vi "Device Level, Display Pulses.vi"(0 "error in":errorcluster, 2 "WFGraph Refnum":refnum<vi>, 3 "waveform":waveform(dbl)={"t0"=timestamp(0 s since 1904-01-01), "dt"=nan, "Y"=[]}, 4 "Zoom (F)":bool) -> (7 "error out":errorcluster, 10 "waveform dup":waveform(dbl)={"t0"=timestamp(3472747248.0780005 s since 1904-01-01), "dt"=nan, "Y"=[]})   [LabVIEW 2010]
doc: "This function zooms in on the first pulse in a pulse train and displays it on Waveform Graph with cursors."
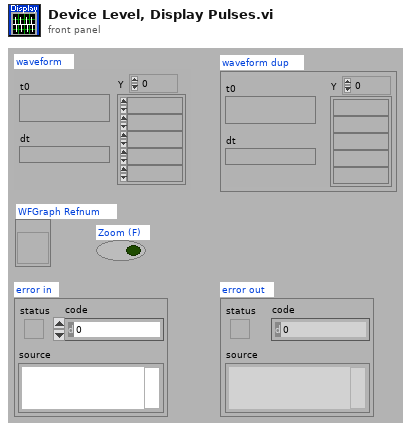
[diagram p1: front panel]
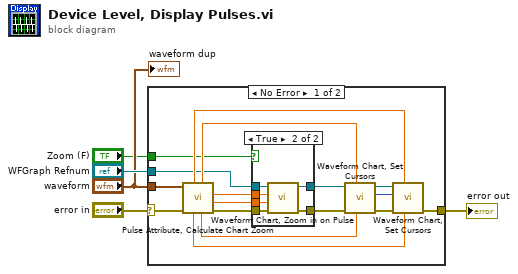
[diagram p0: block diagram]
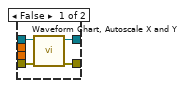
[diagram p2: hidden frame]
diagram:
  n1 = case shown="No Error" "error in" {
    selector: "error in" -> [w19 w33]
    tunnel: "waveform" -> [w18 _]
    tunnel: [w12 w33] -> w5
    tunnel: "WFGraph Refnum" -> [w7 _]
    tunnel: "Zoom (F)" -> [w6 _]
    frame No Error {
      n2 = call "Pulse Attribute, Calculate Chart Zoom.vi"("error in"=w19, "waveform"=w18) -> ("error out"=w22:errorcluster, "X Scale:Max"=w21:dbl, "X Scale:Min"=w20:dbl, "Stim Amp (V)"=w10:dbl, "Stim Trigger (s)"=w16:dbl, "Recvy Amp (V)"=w9:dbl, "Recvy Trigger (s)"=w8:dbl)  [unwired: 2 in, 1 out]
      n3 = case shown="True" w6 {
        tunnel: w22 -> [w26 w32]
        tunnel: w21 -> [_ w31]
        tunnel: w20 -> [_ w30]
        tunnel: w7 -> [w23 w29]
        tunnel: [w25 w28] -> w17
        tunnel: [w24 w27] -> w15
        frame False {
          n4 = call "Waveform Chart, Autoscale X and Y.vi"("error in"=w26, "WFGraph ref"=w23) -> ("error out"=w25:errorcluster, "WFGraph ref dup"=w24:refnum<vi>)  [unwired: 8 in]
        }
        frame True {
          n5 = call "Waveform Chart, Zoom in on Pulse.vi"("error in"=w32, "XScale:Max"=w31, "XScale:Min"=w30, "WFGraph ref"=w29) -> ("error out"=w28:errorcluster, "WFGraph ref dup"=w27:refnum<vi>)  [unwired: 6 in]
        }
      }
      n6 = call "Waveform Chart, Set Cursors.vi"("PosY"=w10, "PosX"=w16, "error in"=w17, "WFGraph ref"=w15) -> ("error out"=w13:errorcluster, "next cursor"=w11:u32, "WFGraph ref dup"=w14:refnum<vi>)  [unwired: 5 in]
      n7 = call "Waveform Chart, Set Cursors.vi"("PosY"=w9, "PosX"=w8, "error in"=w13, "cursor"=w11, "WFGraph ref"=w14) -> ("error out"=w12:errorcluster)  [unwired: 4 in, 2 out]
    }
    frame Error {
    }
  }
  "error out" <- w5
  "waveform dup" <- "waveform"
